vi "SetDbcDataToTreeControl.vi"(7 "에러 입력(에러 없음)":errorcluster, 9 "Open DBC":refnum<k21>, 10 "TreeControl 입력":refnum<vi>) -> (0 "에러 출력":errorcluster)   [LabVIEW 2018, in "Library-Ctrl.lvlib"]
uses:
  Library-Ctrl.lvlib
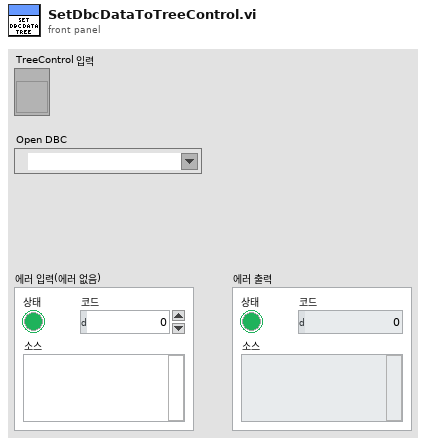
[diagram p1: front panel]
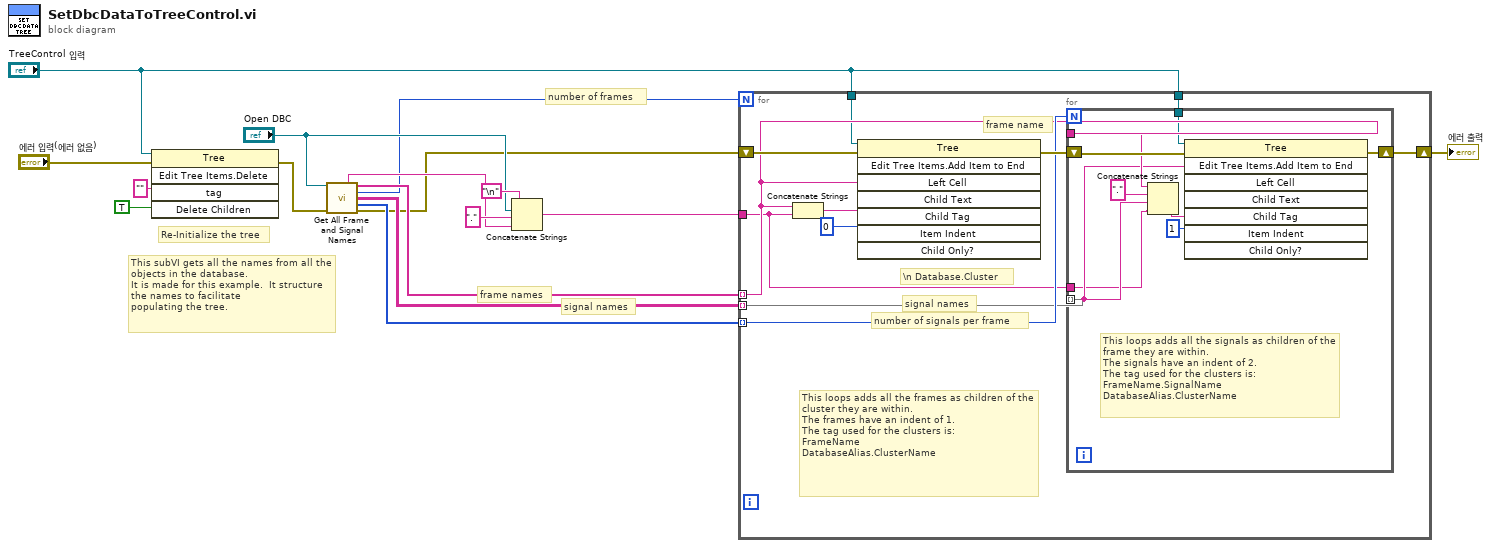
[diagram p0: block diagram]
diagram:
  # "number of frames"
  # "signal names"
  # "frame names"
  # "This subVI gets all the names from all the objects in the database.\nIt is made for this example.  It structure the names to facilitate\npopulating the tree."
  # "Re-Initialize the tree"
  n1 = invoke on="인보크 노드" class="Tree" method="Edit Tree Items.Delete"(reference="TreeControl 입력", error in="에러 입력(에러 없음)", "tag"="" ("Tag"), "Delete Children"=TRUE ("Delete Children?")) -> (error out=w2:errorcluster)  [unwired: 1 in, 4 out]
  n2 = call "Get All Frame and Signal Names.vi"("XNET Cluster"="Open DBC", "error in"=w2) -> ("Cluster"=w7:string, "Frame Names"=w6:string[], "Number of Frames"=w5:i32, "Signal Names"=w4:string[][], "Number of Signals"=w3:i32[], "error out"=w1:errorcluster)  [unwired: 8 in]
  n3 = Concatenate Strings("\n", "Open DBC", "." ("string"), w7) -> (w16:string)
  n4 = for {
    N: w5 -> [_]
    tunnel: w6 -> [w21] mode=indexing
    tunnel: w3 -> [w23] mode=indexing
    tunnel: w4 -> [w22] mode=indexing
    shift-right: [w26] -> w11
    shift-left: w1 -> [w25]
    tunnel: w16 -> [w19]
    tunnel: "TreeControl 입력" -> [w18]
    tunnel: "TreeControl 입력" -> [w17]
    # "\\n Database.Cluster"
    # "signal names"
    # "number of signals per frame"
    # "frame name"
    # "This loops adds all the frames as children of the cluster they are within.\nThe frames have an indent of 1.\nThe tag used for the clusters is: \nFrameName\nDatabaseAlias.ClusterName"
    n5 = Concatenate Strings(w21, w19) -> (w20:string)
    n6 = invoke on="인보크 노드" class="Tree" method="Edit Tree Items.Add Item to End"(reference=w18, error in=w25, "Left Cell"=w21, "Child Tag"=w20, "Item Indent"=0 ("New Item Indentation")) -> (error out=w24:errorcluster)  [unwired: 3 in, 7 out]
    n7 = for {
      N: w23 -> [_]
      tunnel: w21 -> [w32]
      tunnel: w22 -> [w30] mode=indexing
      shift-right: [w36] -> w26
      shift-left: w24 -> [w34]
      tunnel: w19 -> [w29]
      tunnel: w17 -> [w28]
      # "This loops adds all the signals as children of the frame they are within.\nThe signals have an indent of 2.\nThe tag used for the clusters is: \nFrameName.SignalName\nDatabaseAlias.ClusterName"
      n8 = Concatenate Strings(w32, "." ("string"), w30, w29) -> (w33:string)
      n9 = invoke on="인보크 노드" class="Tree" method="Edit Tree Items.Add Item to End"(reference=w28, error in=w34, "Left Cell"=w30, "Child Tag"=w33, "Item Indent"=1 ("New Item Indentation")) -> (error out=w36:errorcluster)  [unwired: 3 in, 7 out]
    }
  }
  "에러 출력" <- w11
